vi "ReadConfig.vi"(8 "error in (no error)":errorcluster, 11 "GRMActor in":refnum<class "StageController.lvclass">) -> (0 "error out":errorcluster, 3 "GRMActor out":refnum<class "StageController.lvclass">)   [LabVIEW 2020, in "StageController.lvlib" / "StageController.lvclass"]
uses:
  StageController.lvclass
  StageController.lvclass/StageController.ctl
  Model/Hardware Abstraction Layer/Component/GenericActor/GenericActor/GenericController.lvclass
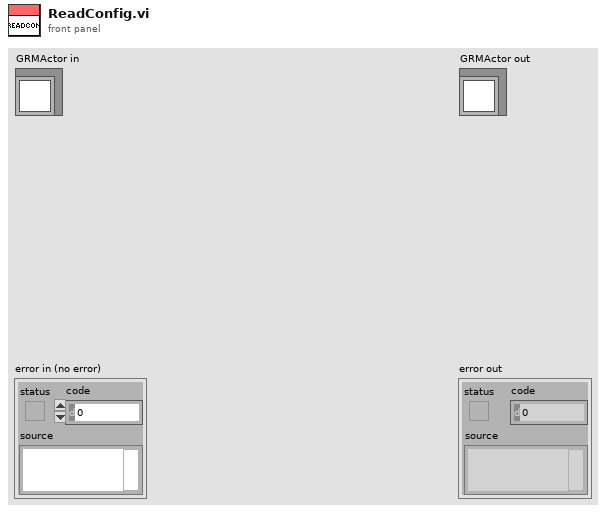
[diagram p1: front panel]
types:
  T1 = typedef "NI_LVConfig.lvlib/Config Data RefNum.ctl" = refnum<k1>
  T2 = cluster{"Values[0]":dbl, "Values[1]":dbl, "Values[2]":dbl, "Values[3]":dbl, "Values[4]":dbl}
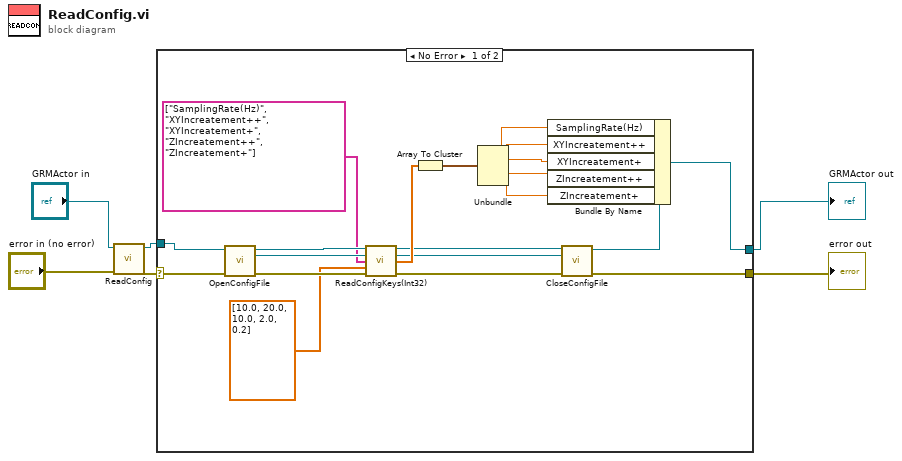
[diagram p0: block diagram]
diagram:
  n1 = call-parent "ReadConfig.vi"("error in (no error)"="error in (no error)", "GRMActor in"="GRMActor in") -> ("error out"=w4:errorcluster, "GRMActor out"=w3:refnum<class "StageController.lvclass">)  [unwired: 8 in]
  n2 = case shown="No Error" w4 {
    selector: w4 -> [w26 w27]
    tunnel: [w18 w27] -> w1
    tunnel: [w21 w28] -> w2
    tunnel: w3 -> [w25 w28]
    frame No Error {
      n3 = call-dynamic "OpenConfigFile.vi"("error in (no error)"=w26, "GRMActor in"=w25) -> ("error out"=w24:errorcluster, "refnum"=w19:T1, "GRMActor out"=w22:refnum<class "StageController.lvclass">)  [unwired: 7 in]
      n4 = call-dynamic "ReadConfigKeys(Int32).vi"("GRMActor in"=w22, "Config Refnum"=w19, "Keys"=string[] ["SamplingRate(Hz)", "XYIncreatement++", "XYIncreatement+", "ZIncreatement++", "ZIncreatement+"] ("Values"), "Default"=dbl[] [10.0, 20.0, 10.0, 2.0, 0.2], "error in (no error)"=w24) -> ("GRMActor out"=w14:refnum<class "StageController.lvclass">, "Config Refnum dup"=w13:T1, "Values"=w16:dbl[], "error out"=w23:errorcluster)  [unwired: 7 in]
      n5 = Array To Cluster(array=w16) -> (cluster=w20:T2)
      n6 = Unbundle(w20) -> ("Values[0]"=w12:dbl, "Values[1]"=w11:dbl, "Values[2]"=w10:dbl, "Values[3]"=w9:dbl, "Values[4]"=w8:dbl)
      n7 = call-dynamic "CloseConfigFile.vi"("error in (no error)"=w23, "refnum"=w13, "GRMActor in"=w14) -> ("error out"=w18:errorcluster, "GRMActor out"=w17:refnum<class "StageController.lvclass">)  [unwired: 7 in]
      n8 = Bundle By Name(cluster=w17, "SamplingRate(Hz)"=w12, "XYIncreatement++"=w11, "XYIncreatement+"=w10, "ZIncreatement++"=w9, "ZIncreatement+"=w8) -> (w21:refnum<class "StageController.lvclass">)
    }
    frame Error {
    }
  }
  "error out" <- w1
  "GRMActor out" <- w2
